vi "setPosition.vi"(0 "reference":refnum<class "RectangularNode.lvclass">, 1 "pos":T1={"x"=nan, "y"=nan} {"y" format="%.2f"; "x" format="%.2f"}, 2 "x":dbl=nan format="%.2f", 3 "y":dbl=nan format="%.2f", 5 "error in (no error)":errorcluster) -> (14 "reference out":refnum<class "RectangularNode.lvclass">, 19 "error out":errorcluster)   [LabVIEW 2016, in "RectangularNode.lvclass"]
doc: "Set the absolute position"
uses:
  <resource>/Framework/Providers/Open_GDS/UML/RectangularNode_class/RectangularNode.lvclass
  <resource>/Framework/Providers/Open_GDS/UML/General/Point/Point Point2D.ctl
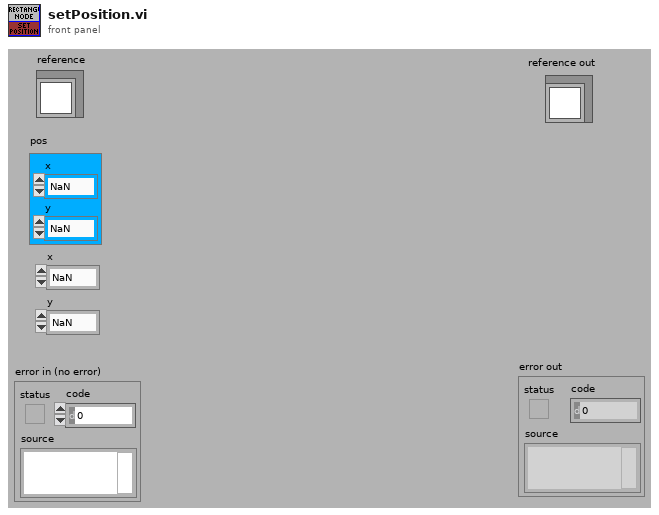
[diagram p1: front panel]
types:
  T1 = typedef "Point Point2D.ctl" = cluster{"x":dbl, "y":dbl}
  T2 = typedef "RectangularNode.lvclass/ObjectAttributes.ctl" = cluster{"bounds":T3}
  T3 = typedef "Rectangle Rectangle2D.ctl" = cluster{"x":dbl, "y":dbl, "width":dbl, "height":dbl}
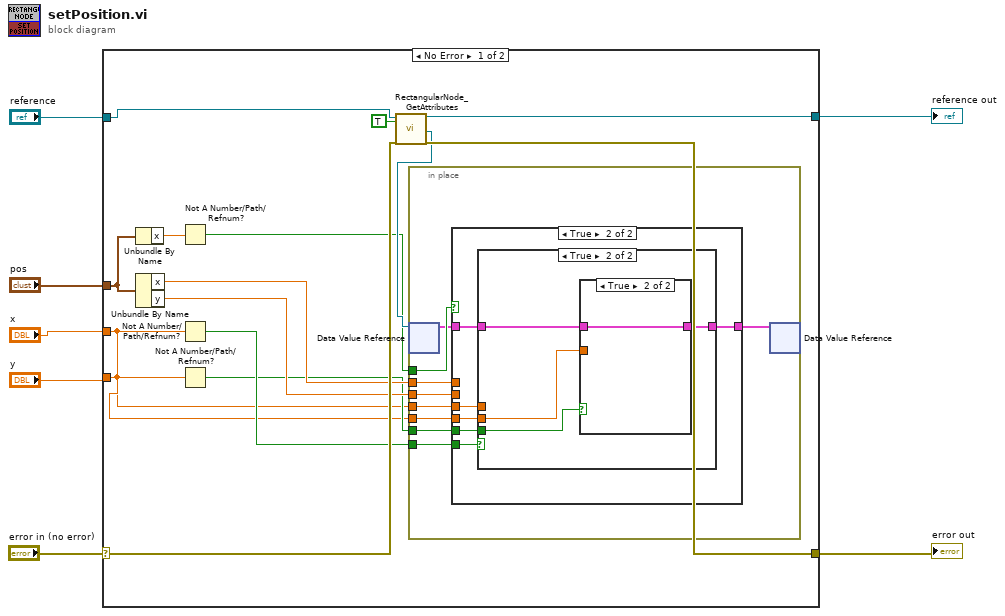
[diagram p0: block diagram]
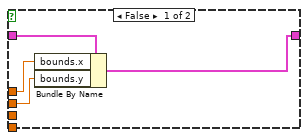
[diagram p2: hidden frame]
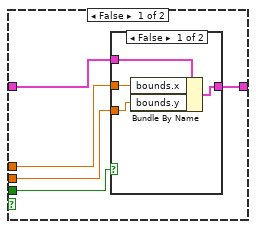
[diagram p3: hidden frame]
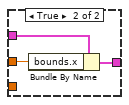
[diagram p4: hidden frame]
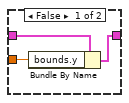
[diagram p5: hidden frame]
diagram:
  n1 = case shown="No Error" "error in (no error)" {
    selector: "error in (no error)" -> [w22 w62]
    tunnel: "reference" -> [w21 w63]
    tunnel: [w20 w62] -> w5
    tunnel: [w19 w63] -> w4
    tunnel: "pos" -> [w17 _]
    tunnel: "x" -> [w8 _]
    tunnel: "y" -> [w9 _]
    frame No Error {
      n2 = Unbundle By Name(w17) -> ("x"=w18:dbl)
      n3 = Unbundle By Name(w17) -> ("x"=w13:dbl, "y"=w12:dbl)
      n4 = Not A Number/Path/Refnum?(number/path/refnum=w18) -> (NaN/Path/Refnum?=w14:bool)
      n5 = Not A Number/Path/Refnum?(number/path/refnum=w8) -> (NaN/Path/Refnum?=w11:bool)
      n6 = Not A Number/Path/Refnum?(number/path/refnum=w9) -> (NaN/Path/Refnum?=w10:bool)
      n7 = call <resource>:"RectangularNode_GetAttributes.vi"("reference in"=w21, "OnlyGetDvrReference(False)"=TRUE, "error in (no error)"=w22) -> ("reference out"=w19:refnum<class "RectangularNode.lvclass">, "DataRef"=w15:refnum<data-value>, "error out"=w20:errorcluster)  [unwired: 13 in, 1 out]
      n8 = in-place {
        in-place-border: w14 -> [w31]
        in-place-border: w13 -> [w29]
        in-place-border: w12 -> [w28]
        in-place-border: w11 -> [w27]
        in-place-border: w10 -> [w26]
        in-place-border: w9 -> [w25]
        in-place-border: w8 -> [w24]
        n9 = in-place-dvr #1(w15) -> (w30:T2)  [unwired: 1 out]
        n10 = case shown="True" w31 {
          tunnel: w30 -> [w35 w41]
          tunnel: [w34 w40] -> w23
          tunnel: w29 -> [w33 _]
          tunnel: w28 -> [w32 _]
          tunnel: w27 -> [_ w39]
          tunnel: w26 -> [_ w38]
          tunnel: w25 -> [_ w37]
          tunnel: w24 -> [_ w36]
          frame False {
            n11 = Bundle By Name(cluster=w35, "bounds.x"=w33, "bounds.y"=w32) -> (w34:T2)
          }
          frame True {
            n12 = case shown="True" w39 {
              tunnel: w41 -> [w45 w57]
              tunnel: [w44 w56] -> w40
              tunnel: w38 -> [w46 w55]
              tunnel: w37 -> [w43 w54]
              tunnel: w36 -> [w42 _]
              frame False {
                n13 = case shown="False" w46 {
                  tunnel: w45 -> [w50 w53]
                  tunnel: [w49 w52] -> w44
                  tunnel: w43 -> [w48 _]
                  tunnel: w42 -> [w47 w51]
                  frame False {
                    n14 = Bundle By Name(cluster=w50, "bounds.x"=w47, "bounds.y"=w48) -> (w49:T2)
                  }
                  frame True {
                    n15 = Bundle By Name(cluster=w53, "bounds.x"=w51) -> (w52:T2)
                  }
                }
              }
              frame True {
                n16 = case shown="True" w55 {
                  tunnel: w57 -> [w60 w61]
                  tunnel: [w59 w61] -> w56
                  tunnel: w54 -> [w58 _]
                  frame False {
                    n17 = Bundle By Name(cluster=w60, "bounds.y"=w58) -> (w59:T2)
                  }
                  frame True {
                  }
                }
              }
            }
          }
        }
        n18 = in-place-dvr #1(w23) -> ()  [unwired: 2 out]
      }
    }
    frame Error {
    }
  }
  "reference out" <- w4
  "error out" <- w5
